vi "DAQ Error.vi"(6 "Chnl Names":string[](array[string]), 8 "error in (no error)":errorcluster, 9 "TDMS File":refnum<k34>, 10 "Task Ref":refnum<k21>, 11 "NI Force Task in":refnum<class "NI Force Task.lvclass">) -> (0 "error out":errorcluster, 3 "NI Force Task out":refnum<class "NI Force Task.lvclass">)   [LabVIEW 2020, in "NI Force Task.lvlib" / "NI Force Task.lvclass"]
uses:
  NI Force Task.lvclass
panel:
  out "Chnl Names 2":string[](array[string])
  out "TDMS File 2":refnum<k34>
  out "Task Ref 2":refnum<k21>
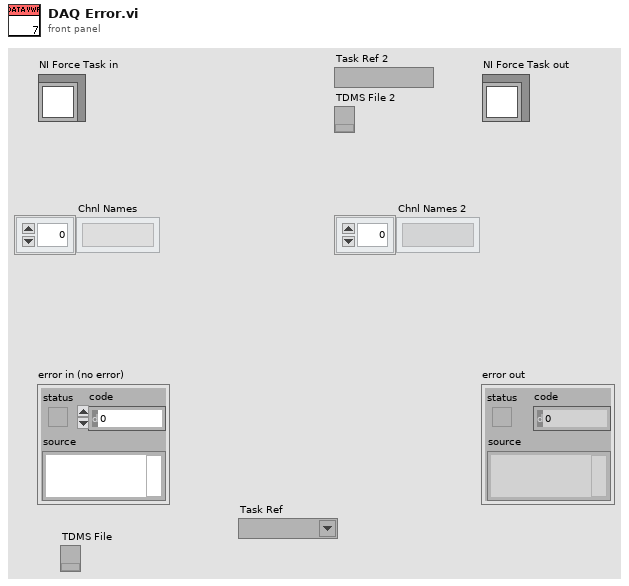
[diagram p1: front panel]
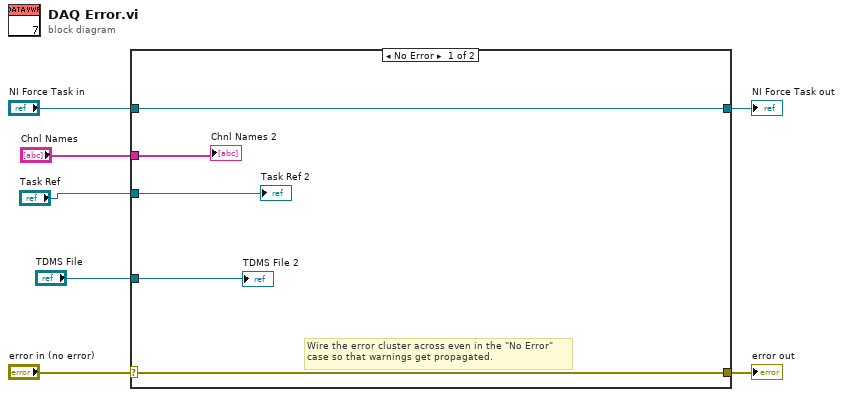
[diagram p0: block diagram]
diagram:
  n1 = case shown="No Error" "error in (no error)" {
    selector: "error in (no error)" -> [w11 w14]
    tunnel: [w11 w14] -> w6
    tunnel: [w12 w13] -> w4
    tunnel: "NI Force Task in" -> [w12 w13]
    tunnel: "Task Ref" -> [w10 _]
    tunnel: "TDMS File" -> [w9 _]
    tunnel: "Chnl Names" -> [w8 _]
    frame No Error {
      # "Wire the error cluster across even in the \"No Error\"\ncase so that warnings get propagated."
      "Task Ref 2" <- w10
      "TDMS File 2" <- w9
      "Chnl Names 2" <- w8
    }
    frame Error {
    }
  }
  "error out" <- w6
  "NI Force Task out" <- w4
